vi "Set Intensity Scales.vi"   [LabVIEW 2016, in "graph_utilities.lvlib"]
uses:
  graph_utilities.lvlib
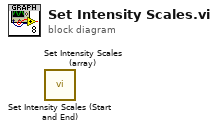
[diagram p0: block diagram]
diagram:
  n1 = call "Set Intensity Scales (Start and End).vi"() -> ()  [unwired: 11 in, 1 out]
  n2 = call "Set Intensity Scales (array).vi"() -> ()  [unwired: 11 in, 1 out]
